vi "CRYResize Panel Child For Load.vi"(8 "spliter array":refnum<vi>[](array[refnum]), 9 "SubPanel array":refnum<vi>[](array[refnum]), 10 "DataView Array Idx":i32) -> ()   [LabVIEW 2013]
uses:
  CRYNew View Global.vi
panel:
  in  "cur_sp_hei":i32
  in  "cur_sp_wid":i32
  in  "cur_sp_ypos":i32
  in  "cur_sp_xpos":i32
  in  "sp_mUp_hei":i32
  in  "sp_mUp_wid":i32
  in  "sp_mUp_ypos":i32
  in  "sp_mUp_xpos":i32
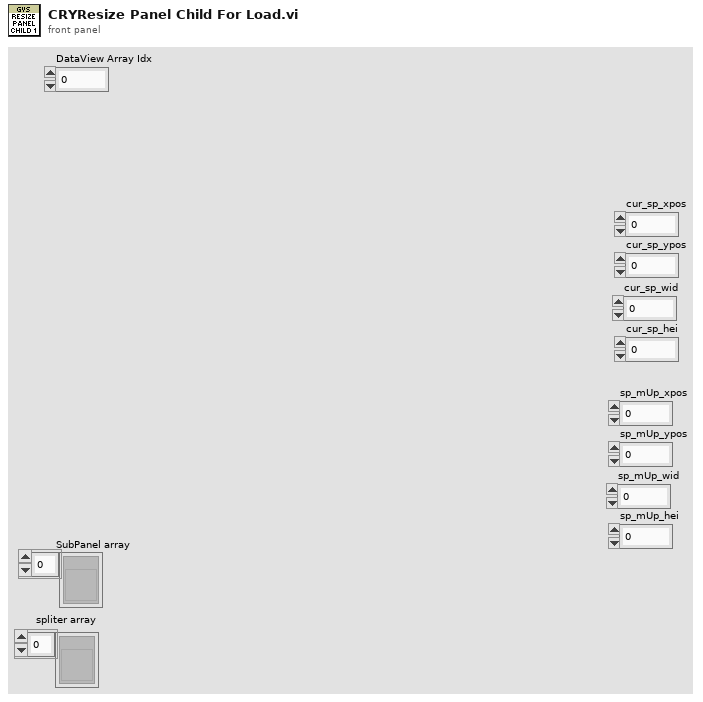
[diagram p1: front panel]
types:
  T1 = typedef "Graph Main Info Cluster.ctl" = cluster{"Selected_BarIdx":i32, "Selected_PanelIdx":i32, "Graph Main VIRef":refnum<vi>, "ToolBarClick":bool, "Spliter Ref Array":refnum<vi>[], "Panel Ref Array":refnum<vi>[], "Spliter_matrix":i32[][], "Panel_matrix":i32[][], "child_spliterIdx_matrix":i32[][], "split_pos_matrix":i32[][], "Title State":bool, "sQueueName":string, "Frame nID":i32, "Graph VIRef Array":cluster{"Graph VIRef":refnum<vi>, "Panel Idx":i32, "Frame VIRef":refnum<vi>, "Icon Ring":i32, "Graph Type":string}[], "View Type":string}
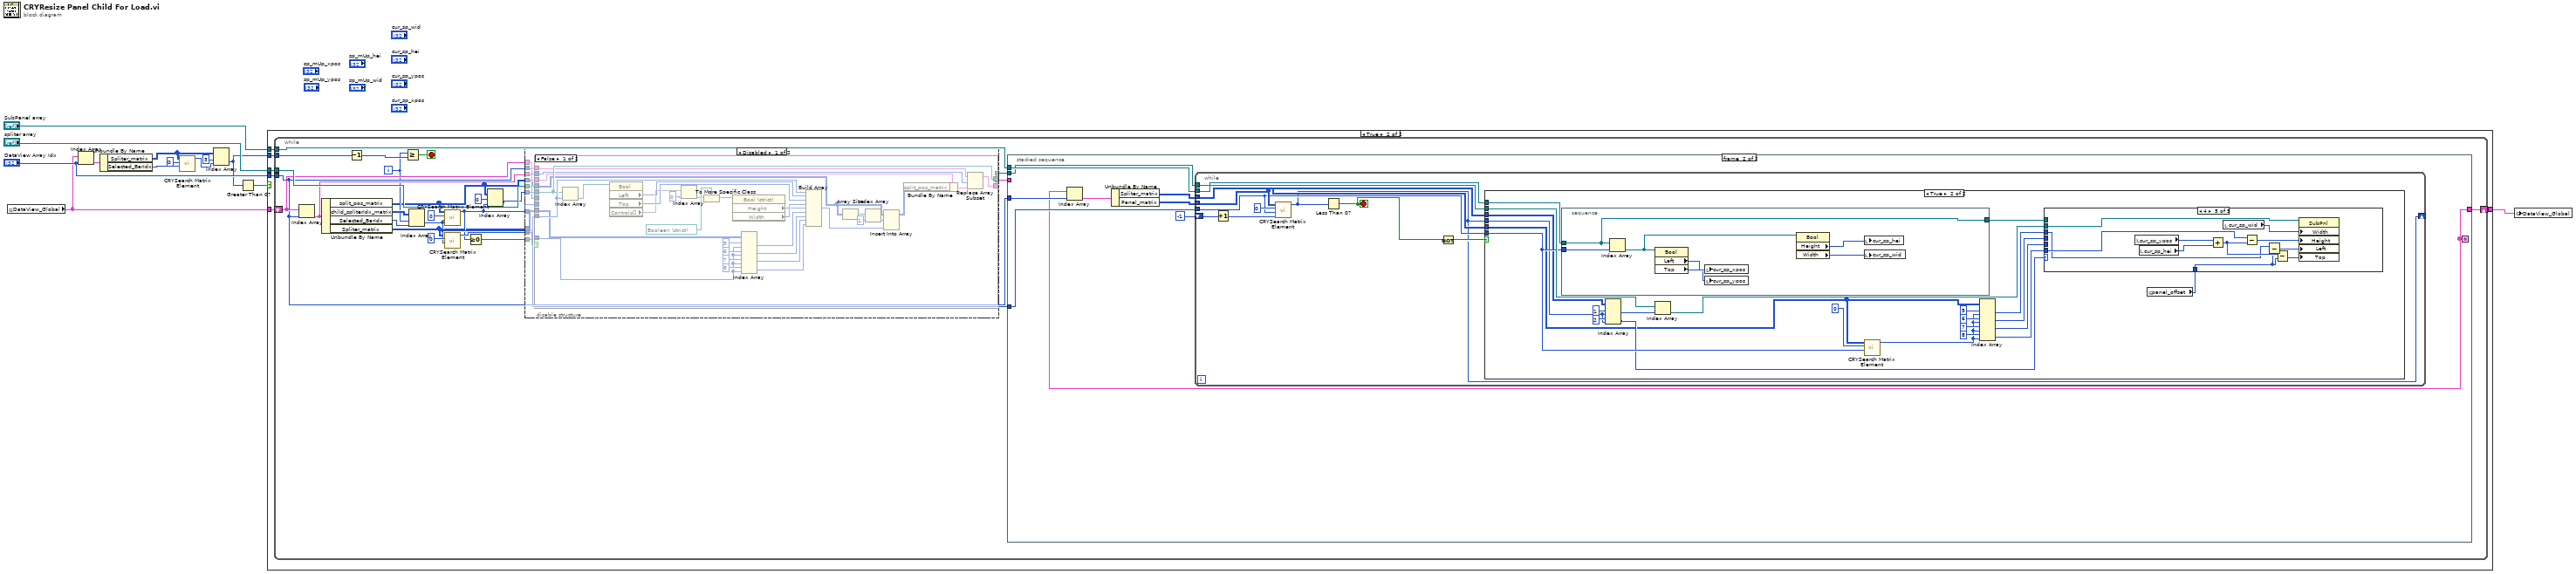
[diagram p0: block diagram]
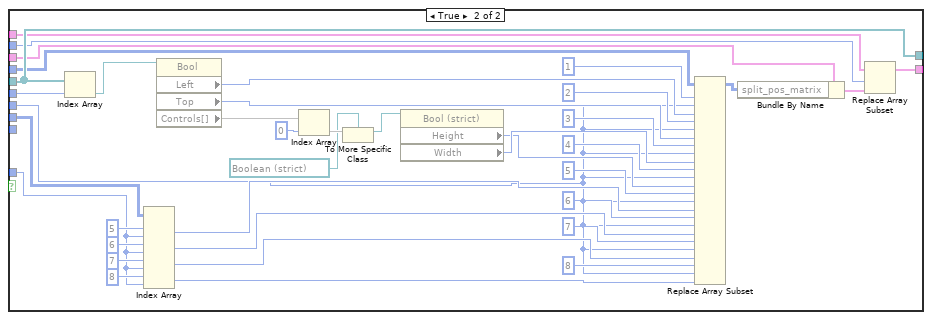
[diagram p3: hidden frame]
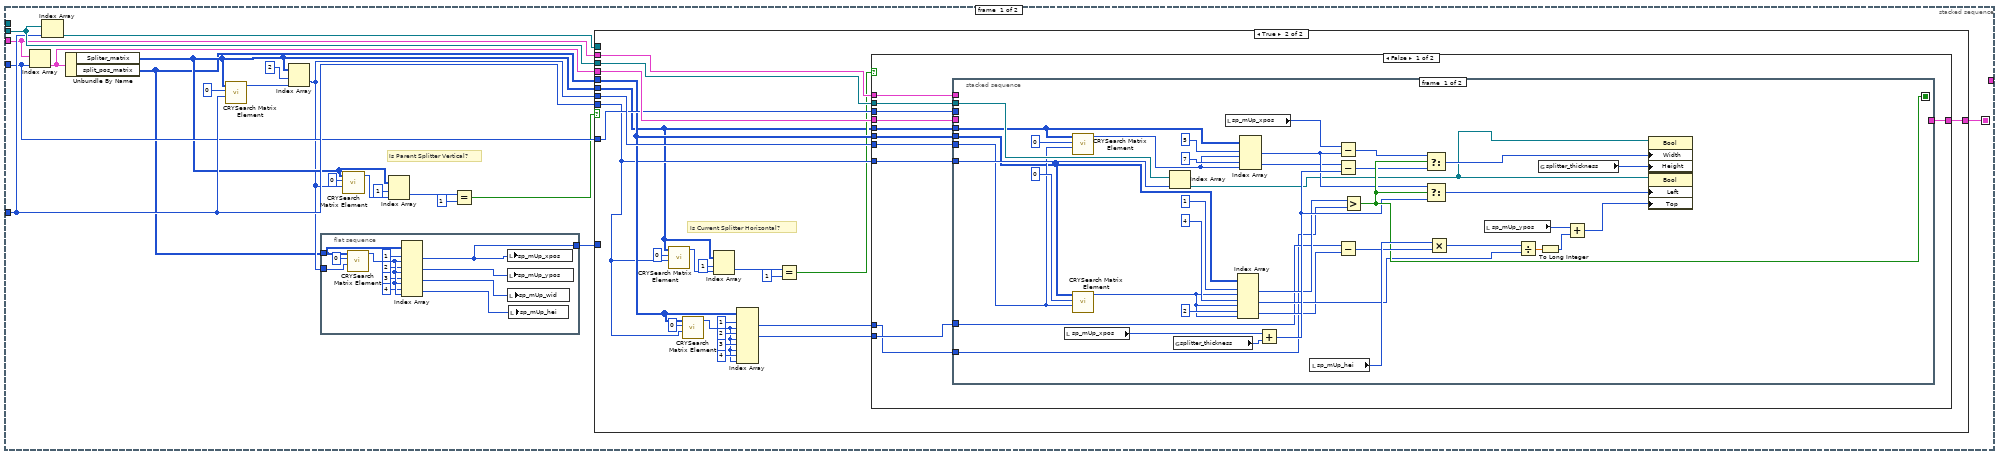
[diagram p5: hidden frame]
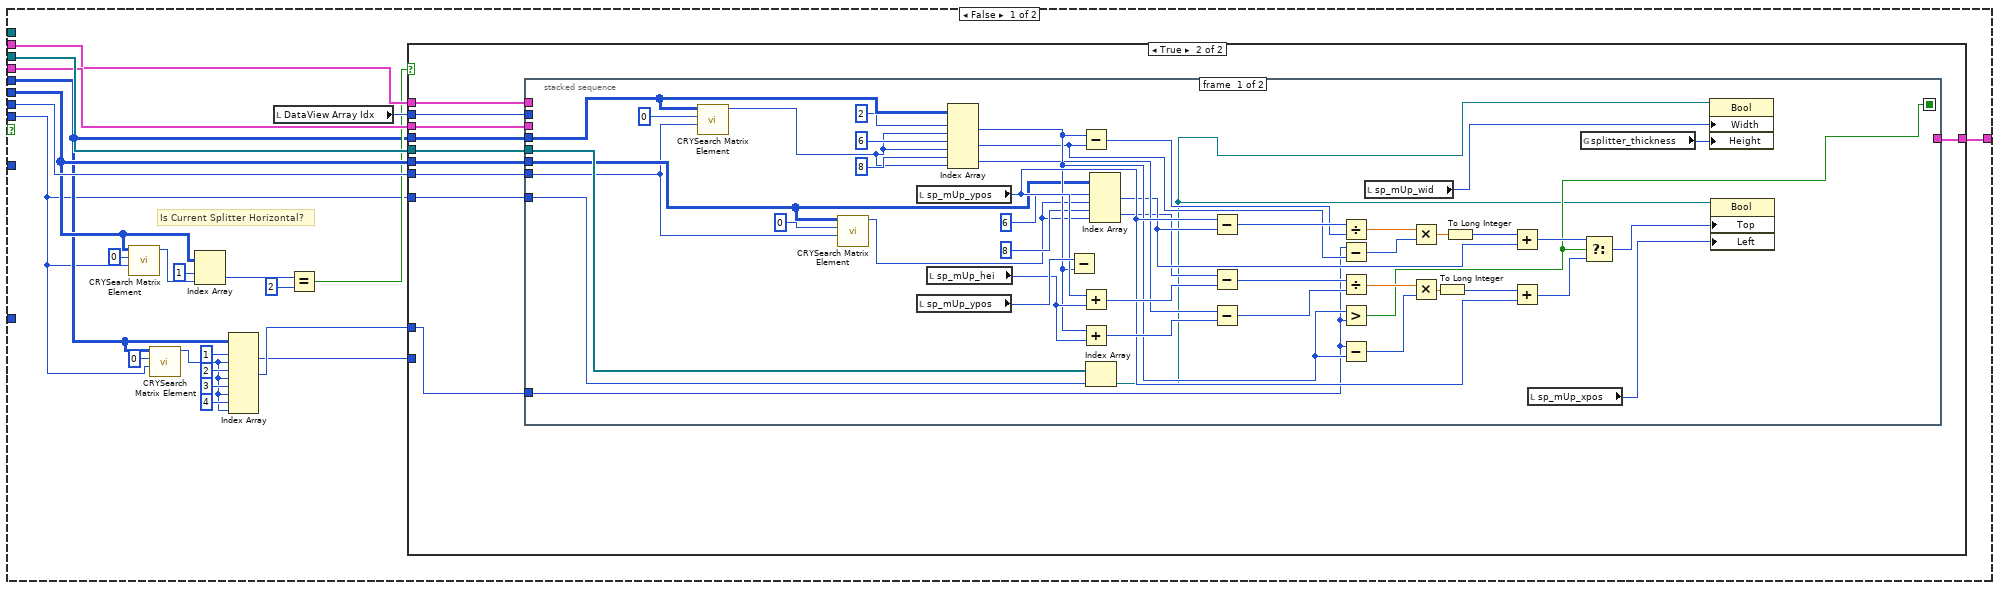
[diagram p6: hidden frame]
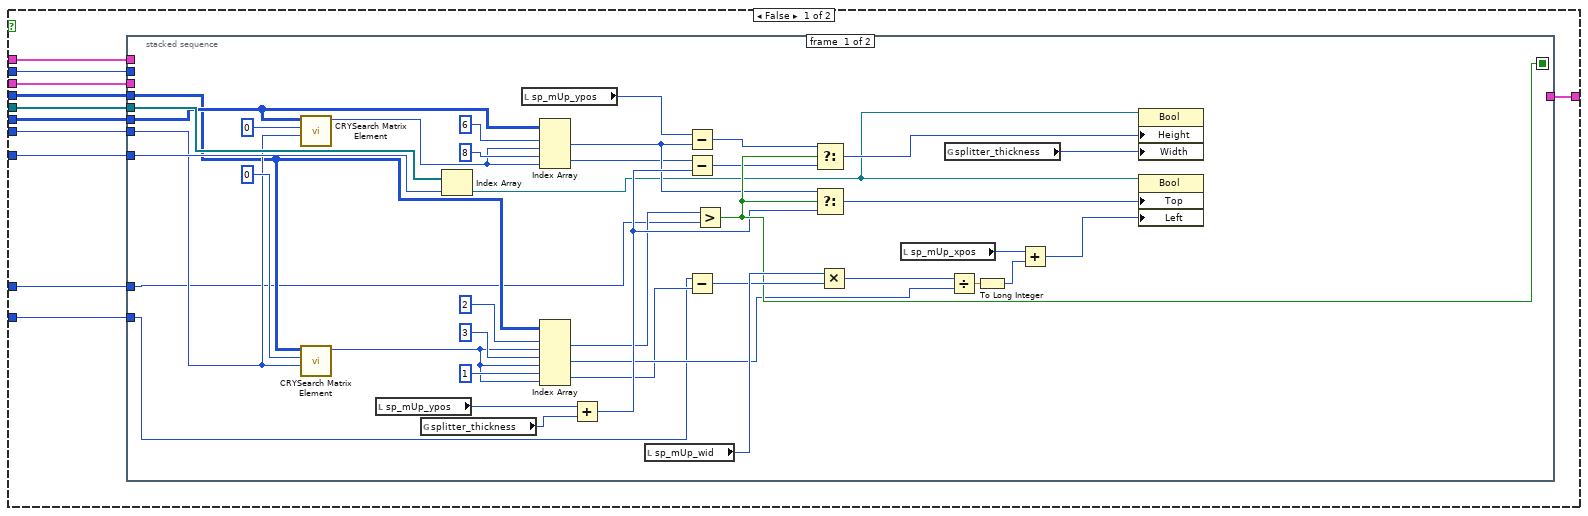
[diagram p7: hidden frame]
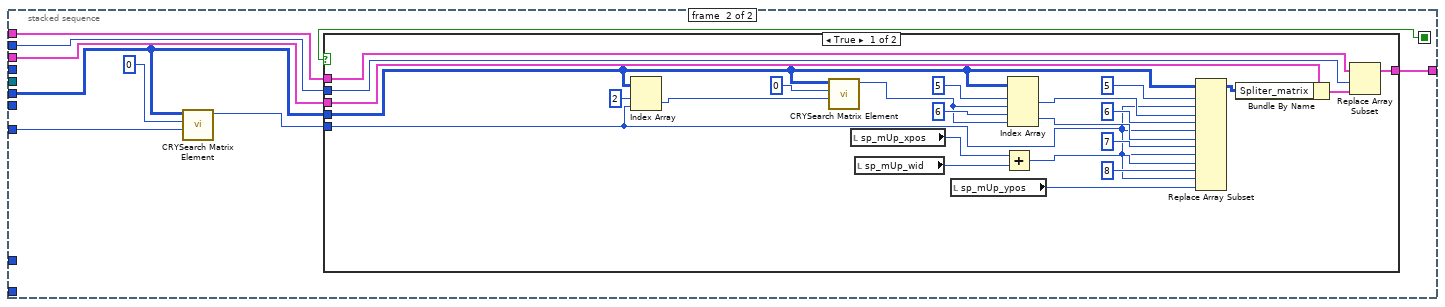
[diagram p8: hidden frame]
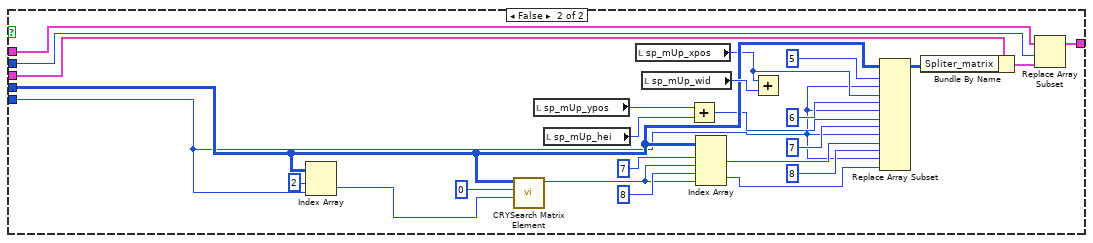
[diagram p9: hidden frame]
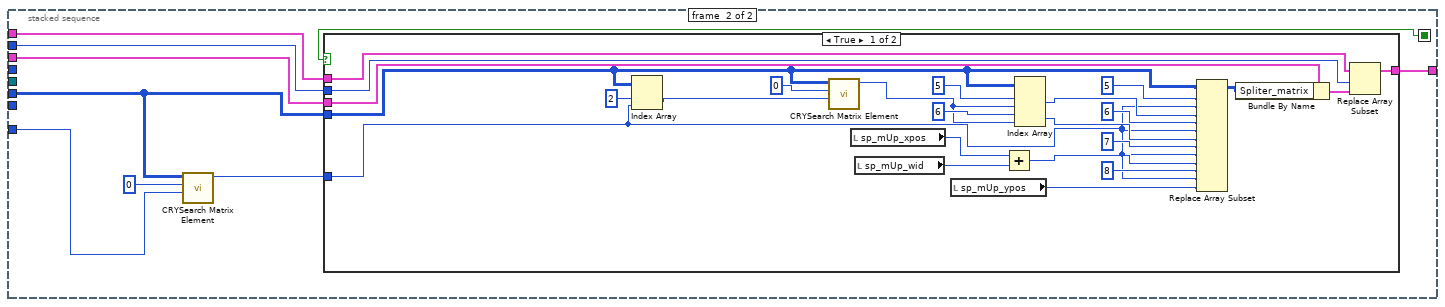
[diagram p10: hidden frame]
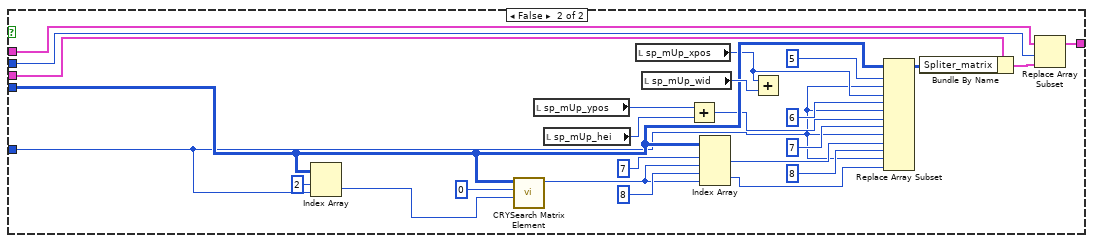
[diagram p11: hidden frame]
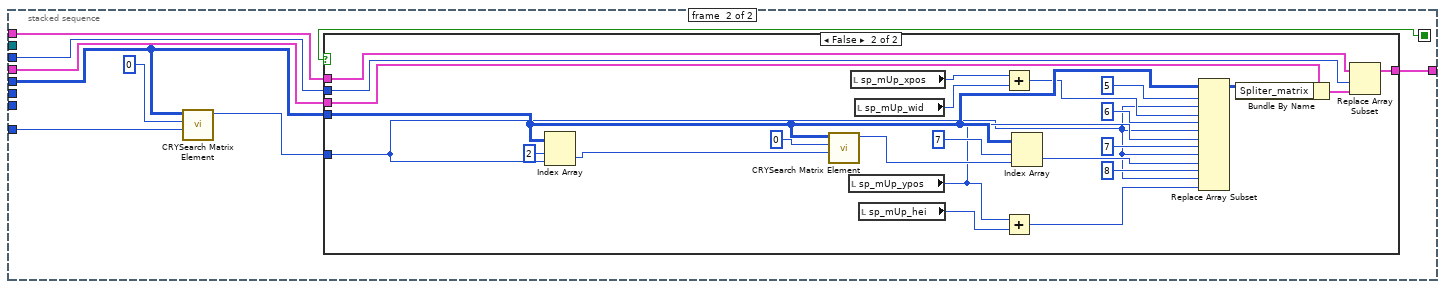
[diagram p12: hidden frame]
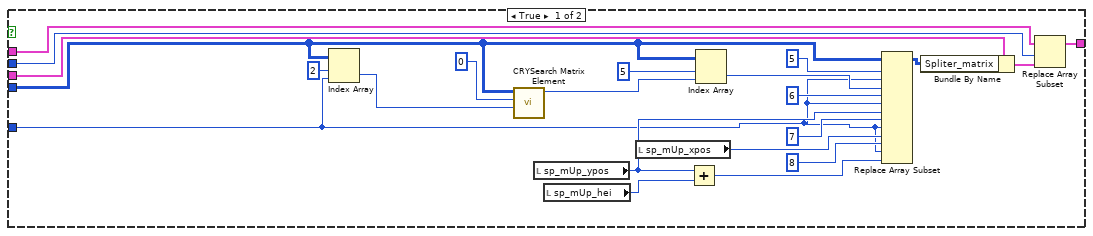
[diagram p13: hidden frame]
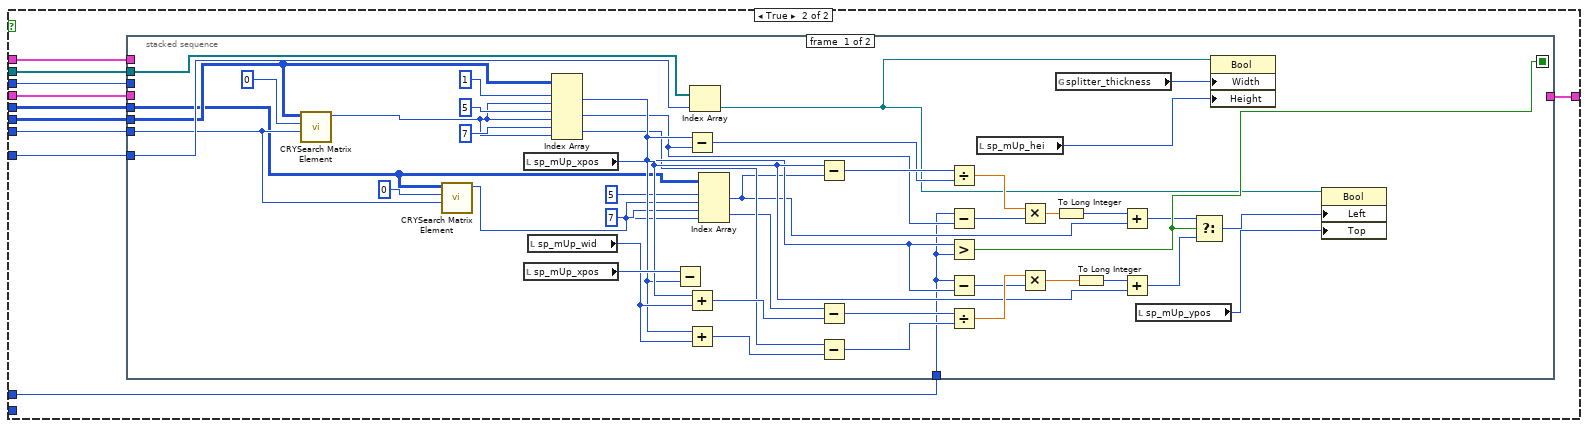
[diagram p14: hidden frame]
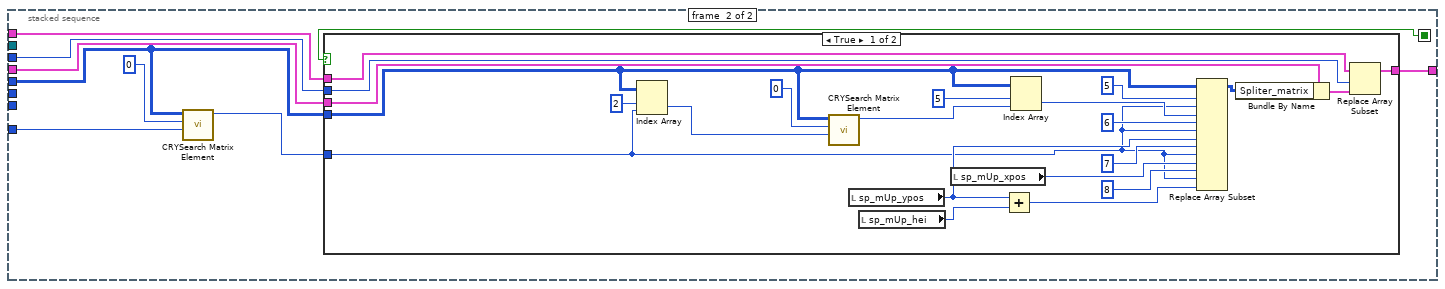
[diagram p15: hidden frame]
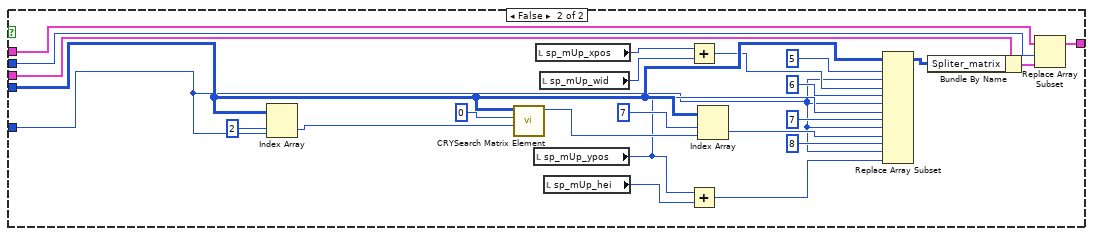
[diagram p16: hidden frame]
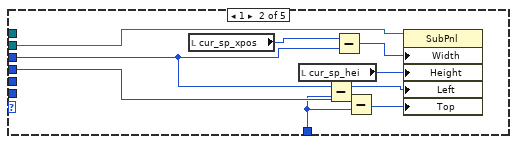
[diagram p19: hidden frame]
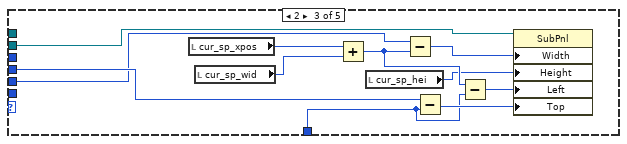
[diagram p20: hidden frame]
diagram:
  n1 = global read "CRYNew View Global.vi" "DataView_Global"() -> (w7:T1[])
  n2 = Index Array(array=w7, index="DataView Array Idx") -> (element=w10:T1)
  n3 = Unbundle By Name(w10) -> ("Spliter_matrix"=w4:i32[][], "Selected_BarIdx"=w9:i32)
  n4 = call "CRYSearch Matrix Element.vi"("element"=w9, "index (row)"=0, "matrix in"=w4) -> ("index of element"=w2:i32)  [unwired: 8 in]
  n5 = Index Array(array=w4, index (row)=3, index (col)=w2) -> (element=w1:i32)
  n6 = Greater Than 0?(x=w1) -> (x > 0?=w5:bool)
  n7 = case shown="True" w5 {
    tunnel: "spliter array" -> [_ w20]
    tunnel: "SubPanel array" -> [_ w19]
    tunnel: "DataView Array Idx" -> [_ w18]
    tunnel: w1 -> [_ w17]
    tunnel: w7 -> [w14 w16]
    tunnel: [w14 w15] -> w6
    frame False {
    }
    frame True {
      n8 = while {
        tunnel: w20 -> [w41]
        tunnel: w17 -> [w30]
        tunnel: w19 -> [w39]
        tunnel: w18 -> [w31]
        shift-right: [w32] -> w15
        shift-left: w16 -> [w34]
        i -> [w28]
        stop <- w42 stop-if-true
        n9 = Index Array(array=w34, index=w31) -> (element=w38:T1)
        n10 = Unbundle By Name(w38) -> ("split_pos_matrix"=w24:i32[][], "child_spliterIdx_matrix"=w29:i32[][], "Selected_BarIdx"=w27:i32, "Spliter_matrix"=w21:i32[][])
        n11 = Decrement(x=w30) -> (x-1=w43:i32)
        n12 = Greater Or Equal?(x=w28, y=w43) -> (x >= y?=w42:bool)
        n13 = Index Array(array=w29, index (row)=w28, index (col)=w27) -> (element=w26:i32)
        n14 = call "CRYSearch Matrix Element.vi"("element"=w26, "index (row)"=0, "matrix in"=w24) -> ("index of element"=w23:i32)  [unwired: 8 in]
        n15 = call "CRYSearch Matrix Element.vi"("element"=w26, "index (row)"=0, "matrix in"=w21) -> ("index of element"=w36:i32)  [unwired: 8 in]
        n16 = Greater Or Equal To 0?(x=w23) -> (x >= 0?=w44:bool)
        n17 = Index Array(array=w24, index (row)=0, index (col)=w23) -> (element=w22:i32)
        n18 = disable-structure shown="Disabled" {
          disable-tunnel: w44 -> [w57 _]
          disable-tunnel: w41 -> [w56 w129]
          disable-tunnel: [w55 w129] -> w40
          disable-tunnel: w38 -> [w54 _]
          disable-tunnel: w36 -> [w53 _]
          disable-tunnel: w34 -> [w52 w130]
          disable-tunnel: [w51 w130] -> w33
          disable-tunnel: w31 -> [w50 _]
          disable-tunnel: w26 -> [w49 _]
          disable-tunnel: w24 -> [w48 _]
          disable-tunnel: w23 -> [w47 _]
          disable-tunnel: w22 -> [w46 _]
          disable-tunnel: w21 -> [w45 _]
          frame Disabled {
            n19 = case shown="False" w57 {
              tunnel: w47 -> [_ w93]
              tunnel: w49 -> [w90 _]
              tunnel: w56 -> [w79 w121]
              tunnel: w46 -> [_ w127]
              tunnel: [w79 w121] -> w55
              tunnel: w53 -> [w69 w110]
              tunnel: w45 -> [w68 w111]
              tunnel: w48 -> [w60 w109]
              tunnel: w50 -> [w77 w119]
              tunnel: w54 -> [w76 w118]
              tunnel: w52 -> [w75 w117]
              tunnel: [w74 w116] -> w51
              frame False {
                n20 = Index Array(array=w79, index=w90) -> (element=w89:refnum<vi>)
                n21 = property class="Bool"(reference=w89) -> ("Left"=w88:i32, "Top"=w87:i32, "Controls[]"=w86)  [unwired: 1 in, 2 out]
                n22 = Index Array(array=w86, index=0) -> (element=w84)
                n23 = To More Specific Class(target class=refnum<vi> refnum ("Boolean"), reference=w84) -> (specific class reference=w82:refnum<vi>)  [unwired: 1 in, 1 out]
                n24 = property class="Bool (strict)"(reference=w82) -> ("Height"=w80:u32, "Width"=w81:u32)  [unwired: 1 in, 2 out]
                n25 = Index Array(array=w68, index (row) #1=5 ("index (row)"), index (col) #1=w69, index (row) #2=6 ("index (row)"), index (col) #2=w69, index (row) #3=7 ("index (row)"), index (col) #3=w69, index (row) #4=8 ("index (row)"), index (col) #4=w69) -> (element #1=w67:i32, element #2=w66:i32, element #3=w65:i32, element #4=w64:i32)
                n26 = Build Array(w90, w88, w87, w81, w80, w67, w66, w65, w64) -> (w59:u32[])
                n27 = Array Size(array=w60) -> (size(s)=w63:i32[])
                n28 = Index Array(array=w63, index=1) -> (element=w61:i32)
                n29 = Insert Into Array(array=w60, index (col)=w61, new element=w59) -> (w58:i32[][])  [unwired: 1 in]
                n30 = Bundle By Name(cluster=w76, "split_pos_matrix"=w58) -> (w78:T1)
                n31 = Replace Array Subset(array=w75, new element=w78, index=w77) -> (w74:T1[])
              }
              frame True {
                n32 = Index Array(array=w121, index=w127) -> (element=w128:refnum<vi>)
                n33 = Index Array(array=w111, index (row) #1=5 ("index (row)"), index (col) #1=w110, index (row) #2=6 ("index (row)"), index (col) #2=w110, index (row) #3=7 ("index (row)"), index (col) #3=w110, index (row) #4=8 ("index (row)"), index (col) #4=w110) -> (element #1=w99:i32, element #2=w97:i32, element #3=w95:i32, element #4=w92:i32)
                n34 = property class="Bool"(reference=w128) -> ("Left"=w107:i32, "Top"=w105:i32, "Controls[]"=w126)  [unwired: 1 in, 2 out]
                n35 = Index Array(array=w126, index=0) -> (element=w124)
                n36 = To More Specific Class(target class=refnum<vi> refnum ("Boolean"), reference=w124) -> (specific class reference=w122:refnum<vi>)  [unwired: 1 in, 1 out]
                n37 = property class="Bool (strict)"(reference=w122) -> ("Height"=w101:u32, "Width"=w103:u32)  [unwired: 1 in, 2 out]
                n38 = Replace Array Subset(array=w109, new element #1=w107, index (row) #1=1 ("disabled index (row)"), index (col) #1=w93, new element #2=w105, index (row) #2=2 ("disabled index (row)"), index (col) #2=w93, new element #3=w103, index (row) #3=3 ("disabled index (row)"), index (col) #3=w93, new element #4=w101, index (row) #4=4 ("disabled index (row)"), index (col) #4=w93, new element #5=w99, index (row) #5=5 ("disabled index (row)"), index (col) #5=w93, new element #6=w97, index (row) #6=6 ("disabled index (row)"), index (col) #6=w93, new element #7=w95, index (row) #7=7 ("disabled index (row)"), index (col) #7=w93, new element #8=w92, index (row) #8=8 ("disabled index (row)"), index (col) #8=w93) -> (w91:i32[][])
                n39 = Bundle By Name(cluster=w118, "split_pos_matrix"=w91) -> (w120:T1)
                n40 = Replace Array Subset(array=w117, new element=w120, index=w119) -> (w116:T1[])
              }
            }
          }
          frame Enabled {
          }
        }
        n41 = stacked-sequence {
          seq-local: [w144 _] -> [_ w645]
          tunnel: w40 -> [w149 w651]
          tunnel: w26 -> [w146 w653]
          tunnel: w39 -> [_ w652]
          tunnel: w31 -> [w143 w648]
          tunnel: w33 -> [w145 _]
          tunnel: [_ w645] -> w32
          frame #0 {
            # "Is Parent Splitter Vertical?"
            n42 = Index Array(array=w145, index=w143) -> (element=w148:T1)
            n43 = Index Array(array=w149, index=w146) -> (element=w150:refnum<vi>)
            n44 = Unbundle By Name(w148) -> ("Spliter_matrix"=w139:i32[][], "split_pos_matrix"=w132:i32[][])
            n45 = call "CRYSearch Matrix Element.vi"("element"=w146, "index (row)"=0, "matrix in"=w139) -> ("index of element"=w141:i32)  [unwired: 8 in]
            n46 = Index Array(array=w139, index (row)=2, index (col)=w141) -> (element=w133:i32)
            n47 = flat-sequence {
              tunnel: w133 -> [w161]
              tunnel: w132 -> [w152]
              tunnel: [w151] -> w131
              frame #0 {
                n48 = call "CRYSearch Matrix Element.vi"("element"=w161, "index (row)"=0, "matrix in"=w152) -> ("index of element"=w160:i32)  [unwired: 8 in]
                n49 = Index Array(array=w152, index (row) #1=1 ("disabled index (row)"), index (col) #1=w160, index (row) #2=2 ("disabled index (row)"), index (col) #2=w160, index (row) #3=3 ("disabled index (row)"), index (col) #3=w160, index (row) #4=4 ("disabled index (row)"), index (col) #4=w160) -> (element #1=w151:i32, element #2=w155:i32, element #3=w154:i32, element #4=w153:i32)
                n50 = local write "sp_mUp_xpos"(w151) -> ()
                n51 = local write "sp_mUp_ypos"(w155) -> ()
                n52 = local write "sp_mUp_wid"(w154) -> ()
                n53 = local write "sp_mUp_hei"(w153) -> ()
              }
            }
            n54 = call "CRYSearch Matrix Element.vi"("element"=w133, "index (row)"=0, "matrix in"=w139) -> ("index of element"=w134:i32)  [unwired: 8 in]
            n55 = Index Array(array=w139, index (row)=1 ("disabled index (row)"), index (col)=w134) -> (element=w137:i32)
            n56 = Equal?(x=w137, y=1) -> (x = y?=w135:bool)
            n57 = case shown="True" w135 {
              tunnel: w150 -> [_ _]
              tunnel: w133 -> [w185 w429]
              tunnel: w149 -> [w184 w428]
              tunnel: w146 -> [w163 w411]
              tunnel: w132 -> [w166 w412]
              tunnel: w139 -> [w174 w407]
              tunnel: w148 -> [w183 w427]
              tunnel: w145 -> [w181 w426]
              tunnel: [w180 w425] -> w144
              tunnel: w143 -> [_ w424]
              tunnel: w131 -> [_ _]
              frame False {
                # "Is Current Splitter Horizontal?"
                n58 = call "CRYSearch Matrix Element.vi"("element"=w163, "index (row)"=0, "matrix in"=w174) -> ("index of element"=w179:i32)  [unwired: 8 in]
                n59 = call "CRYSearch Matrix Element.vi"("element"=w163, "index (row)"=0, "matrix in"=w166) -> ("index of element"=w168:i32)  [unwired: 8 in]
                n60 = Index Array(array=w174, index (row)=1 ("disabled index (row)"), index (col)=w179) -> (element=w177:i32)
                n61 = Index Array(array=w166, index (row) #1=1 ("disabled index (row)"), index (col) #1=w168, index (row) #2=2 ("disabled index (row)"), index (col) #2=w168, index (row) #3=3 ("disabled index (row)"), index (col) #3=w168, index (row) #4=4 ("disabled index (row)"), index (col) #4=w168) -> (element #1=w164:i32, element #2=w165:i32)  [unwired: 2 out]
                n62 = local read "DataView Array Idx"() -> (w182:i32)
                n63 = Equal?(x=w177, y=2) -> (x = y?=w173:bool)
                n64 = case shown="True" w173 {
                  tunnel: w185 -> [w194 w301]
                  tunnel: w184 -> [w196 w302]
                  tunnel: w163 -> [w195 w303]
                  tunnel: w166 -> [w193 w300]
                  tunnel: w174 -> [w192 w299]
                  tunnel: w183 -> [w191 w298]
                  tunnel: w182 -> [w190 w297]
                  tunnel: w181 -> [w189 w296]
                  tunnel: [w188 w295] -> w180
                  tunnel: w165 -> [w187 w294]
                  tunnel: w164 -> [w186 _]
                  frame False {
                    n65 = stacked-sequence {
                      seq-local: [w224 _] -> [_ w244]
                      tunnel: w196 -> [w235 _]
                      tunnel: w195 -> [w234 w239]
                      tunnel: w194 -> [w217 _]
                      tunnel: w193 -> [w210 _]
                      tunnel: w192 -> [w216 w241]
                      tunnel: w191 -> [_ w243]
                      tunnel: w190 -> [_ w242]
                      tunnel: w189 -> [_ w237]
                      tunnel: [_ w236] -> w188
                      tunnel: w187 -> [w202 _]
                      tunnel: w186 -> [w201 _]
                      frame #0 {
                        n66 = call "CRYSearch Matrix Element.vi"("element"=w217, "index (row)"=0, "matrix in"=w216) -> ("index of element"=w213:i32)  [unwired: 8 in]
                        n67 = call "CRYSearch Matrix Element.vi"("element"=w217, "index (row)"=0, "matrix in"=w210) -> ("index of element"=w206:i32)  [unwired: 8 in]
                        n68 = local read "sp_mUp_ypos"() -> (w233:i32)
                        n69 = global read "CRYNew View Global.vi" "splitter_thickness"() -> (w197:u32)
                        n70 = Index Array(array=w235, index=w234) -> (element=w200:refnum<vi>)
                        n71 = local read "sp_mUp_ypos"() -> (w223:i32)
                        n72 = Index Array(array=w216, index (row) #1=6 ("index (row)"), index (col) #1=w213, index (row) #2=8 ("index (row)"), index (col) #2=w213) -> (element #1=w212:i32, element #2=w211:i32)
                        n73 = Index Array(array=w210, index (row) #1=2 ("index (row)"), index (col) #1=w206, index (row) #2=3 ("index (row)"), index (col) #2=w206, index (row) #3=1 ("index (row)"), index (col) #3=w206) -> (element #1=w205:i32, element #2=w204:i32, element #3=w203:i32)
                        n74 = Add(x=w233, y=w197) -> (x+y=w221:u32)
                        n75 = local read "sp_mUp_wid"() -> (w230:i32)
                        n76 = Subtract(x=w223, y=w212) -> (x-y=w222:i32)
                        n77 = Subtract(x=w211, y=w221) -> (x-y=w220:u32)
                        n78 = Subtract(x=w201, y=w203) -> (x-y=w225:i32)
                        n79 = Greater?(x=w205, y=w202) -> (0:w224:bool)
                        n80 = Select(t=w222, s=w224, f=w220) -> (s? t:f=w231:u32)
                        n81 = Select(t=w212, s=w224, f=w221) -> (s? t:f=w232:u32)
                        n82 = Multiply(x=w230, y=w225) -> (x*y=w229:i32)
                        n83 = local read "sp_mUp_xpos"() -> (w228:i32)
                        n84 = global read "CRYNew View Global.vi" "splitter_thickness"() -> (w199:u32)
                        n85 = Divide(x=w229, y=w204) -> (x/y=w227:dbl)
                        n86 = To Long Integer(number=w227) -> (32bit integer=w198:i32)
                        n87 = Add(x=w228, y=w198) -> (x+y=w226:i32)
                        n88 = property class="Bool"(reference=w200, "Height"=w231, "Width"=w199) -> ()  [unwired: 1 in, 2 out]
                        n89 = property class="Bool"(reference=w200, "Top"=w232, "Left"=w226) -> ()  [unwired: 1 in, 2 out]
                      }
                      frame #1 {
                        n90 = call "CRYSearch Matrix Element.vi"("element"=w239, "index (row)"=0, "matrix in"=w241) -> ("index of element"=w238:i32)  [unwired: 8 in]
                        n91 = case shown="True" w244 {
                          tunnel: w238 -> [w247 w271]
                          tunnel: w241 -> [w255 w279]
                          tunnel: w243 -> [w265 w289]
                          tunnel: w242 -> [w264 w288]
                          tunnel: w237 -> [w262 w286]
                          tunnel: [w261 w285] -> w236
                          frame True {
                            n92 = Index Array(array=w255, index (row)=2, index (col)=w247) -> (element=w259:i32)
                            n93 = call "CRYSearch Matrix Element.vi"("element"=w259, "index (row)"=0, "matrix in"=w255) -> ("index of element"=w256:i32)  [unwired: 8 in]
                            n94 = local read "sp_mUp_xpos"() -> (w267:i32)
                            n95 = local read "sp_mUp_wid"() -> (w268:i32)
                            n96 = local read "sp_mUp_ypos"() -> (w246:i32)
                            n97 = Add(x=w267, y=w268) -> (x+y=w249:i32)
                            n98 = Index Array(array=w255, index (row) #1=5 ("index (row)"), index (col) #1=w256, index (row) #2=6 ("index (row)"), index (col) #2=w256) -> (element #1=w253:i32, element #2=w251:i32)
                            n99 = Replace Array Subset(array=w255, new element #1=w253, index (row) #1=5 ("disabled index (row)"), index (col) #1=w247, new element #2=w251, index (row) #2=6 ("disabled index (row)"), index (col) #2=w247, new element #3=w249, index (row) #3=7 ("disabled index (row)"), index (col) #3=w247, new element #4=w246, index (row) #4=8 ("disabled index (row)"), index (col) #4=w247) -> (w245:i32[][])
                            n100 = Bundle By Name(cluster=w265, "Spliter_matrix"=w245) -> (w266:T1)
                            n101 = Replace Array Subset(array=w262, new element=w266, index=w264) -> (w261:T1[])
                          }
                          frame False {
                            n102 = Index Array(array=w279, index (row)=2, index (col)=w271) -> (element=w283:i32)
                            n103 = call "CRYSearch Matrix Element.vi"("element"=w283, "index (row)"=0, "matrix in"=w279) -> ("index of element"=w280:i32)  [unwired: 8 in]
                            n104 = local read "sp_mUp_ypos"() -> (w292:i32)
                            n105 = local read "sp_mUp_hei"() -> (w293:i32)
                            n106 = local read "sp_mUp_xpos"() -> (w277:i32)
                            n107 = local read "sp_mUp_wid"() -> (w291:i32)
                            n108 = Add(x=w292, y=w293) -> (x+y=w275:i32)
                            n109 = Index Array(array=w279, index (row) #1=7 ("index (row)"), index (col) #1=w280, index (row) #2=8 ("index (row)"), index (col) #2=w280) -> (element #1=w273:i32, element #2=w270:i32)
                            n110 = Add(x=w277, y=w291) -> ()  [unwired: 1 out]
                            n111 = Replace Array Subset(array=w279, new element #1=w277, index (row) #1=5 ("disabled index (row)"), index (col) #1=w271, new element #2=w275, index (row) #2=6 ("disabled index (row)"), index (col) #2=w271, new element #3=w273, index (row) #3=7 ("disabled index (row)"), index (col) #3=w271, new element #4=w270, index (row) #4=8 ("disabled index (row)"), index (col) #4=w271) -> (w269:i32[][])
                            n112 = Bundle By Name(cluster=w289, "Spliter_matrix"=w269) -> (w290:T1)
                            n113 = Replace Array Subset(array=w286, new element=w290, index=w288) -> (w285:T1[])
                          }
                        }
                      }
                    }
                  }
                  frame True {
                    n114 = stacked-sequence {
                      seq-local: [w327 _] -> [_ w357]
                      tunnel: w303 -> [w310 w353]
                      tunnel: w302 -> [w347 _]
                      tunnel: w301 -> [w308 _]
                      tunnel: w300 -> [w324 _]
                      tunnel: w299 -> [w316 w352]
                      tunnel: w298 -> [_ w356]
                      tunnel: w297 -> [_ w355]
                      tunnel: w296 -> [_ w350]
                      tunnel: [_ w349] -> w295
                      tunnel: w294 -> [w309 _]
                      frame #0 {
                        n115 = call "CRYSearch Matrix Element.vi"("element"=w308, "index (row)"=0, "matrix in"=w324) -> ("index of element"=w320:i32)  [unwired: 8 in]
                        n116 = call "CRYSearch Matrix Element.vi"("element"=w308, "index (row)"=0, "matrix in"=w316) -> ("index of element"=w313:i32)  [unwired: 8 in]
                        n117 = local read "sp_mUp_ypos"() -> (w331:i32)
                        n118 = local read "sp_mUp_ypos"() -> (w348:i32)
                        n119 = local read "sp_mUp_hei"() -> (w344:i32)
                        n120 = Index Array(array=w324, index (row) #1=2 ("index (row)"), index (col) #1=w320, index (row) #2=6 ("index (row)"), index (col) #2=w320, index (row) #3=8 ("index (row)"), index (col) #3=w320) -> (element #1=w319:i32, element #2=w318:i32, element #3=w317:i32)
                        n121 = Subtract(x=w348, y=w319) -> ()  [unwired: 1 out]
                        n122 = Subtract(x=w319, y=w318) -> (x-y=w338:i32)
                        n123 = Add(x=w331, y=w344) -> (x+y=w332:i32)
                        n124 = Add(x=w319, y=w344) -> (x+y=w333:i32)
                        n125 = Index Array(array=w347, index=w310) -> (element=w307:refnum<vi>)
                        n126 = Index Array(array=w316, index (row) #1=6 ("index (row)"), index (col) #1=w313, index (row) #2=8 ("index (row)"), index (col) #2=w313) -> (element #1=w312:i32, element #2=w311:i32)
                        n127 = Subtract(x=w331, y=w312) -> (x-y=w339:i32)
                        n128 = Subtract(x=w311, y=w332) -> (x-y=w343:i32)
                        n129 = Subtract(x=w317, y=w333) -> (x-y=w342:i32)
                        n130 = Divide(x=w339, y=w338) -> (x/y=w337:dbl)
                        n131 = Subtract(x=w309, y=w318) -> (x-y=w336:i32)
                        n132 = Divide(x=w343, y=w342) -> (x/y=w341:dbl)
                        n133 = Greater?(x=w319, y=w309) -> (0:w327:bool)
                        n134 = Subtract(x=w309, y=w319) -> (x-y=w334:i32)
                        n135 = local read "sp_mUp_wid"() -> (w346:i32)
                        n136 = Multiply(x=w337, y=w336) -> (x*y=w335:dbl)
                        n137 = Multiply(x=w341, y=w334) -> (x*y=w340:dbl)
                        n138 = To Long Integer(number=w340) -> (32bit integer=w305:i32)
                        n139 = To Long Integer(number=w335) -> (32bit integer=w306:i32)
                        n140 = Add(x=w306, y=w312) -> (x+y=w330:i32)
                        n141 = Add(x=w305, y=w331) -> (x+y=w329:i32)
                        n142 = local read "sp_mUp_xpos"() -> (w345:i32)
                        n143 = global read "CRYNew View Global.vi" "splitter_thickness"() -> (w304:u32)
                        n144 = Select(t=w330, s=w327, f=w329) -> (s? t:f=w328:i32)
                        n145 = property class="Bool"(reference=w307, "Width"=w346, "Height"=w304) -> ()  [unwired: 1 in, 2 out]
                        n146 = property class="Bool"(reference=w307, "Top"=w328, "Left"=w345) -> ()  [unwired: 1 in, 2 out]
                      }
                      frame #1 {
                        n147 = call "CRYSearch Matrix Element.vi"("element"=w353, "index (row)"=0, "matrix in"=w352) -> ("index of element"=w351:i32)  [unwired: 8 in]
                        n148 = case shown="True" w357 {
                          tunnel: w351 -> [w359 w383]
                          tunnel: w352 -> [w368 w392]
                          tunnel: w356 -> [w378 w402]
                          tunnel: w355 -> [w377 w401]
                          tunnel: w350 -> [w375 w399]
                          tunnel: [w374 w398] -> w349
                          frame True {
                            n149 = Index Array(array=w368, index (row)=2, index (col)=w359) -> (element=w373:i32)
                            n150 = call "CRYSearch Matrix Element.vi"("element"=w373, "index (row)"=0, "matrix in"=w368) -> ("index of element"=w369:i32)  [unwired: 8 in]
                            n151 = local read "sp_mUp_xpos"() -> (w380:i32)
                            n152 = local read "sp_mUp_wid"() -> (w381:i32)
                            n153 = local read "sp_mUp_ypos"() -> (w358:i32)
                            n154 = Add(x=w380, y=w381) -> (x+y=w361:i32)
                            n155 = Index Array(array=w368, index (row) #1=5 ("index (row)"), index (col) #1=w369, index (row) #2=6 ("index (row)"), index (col) #2=w369) -> (element #1=w365:i32, element #2=w363:i32)
                            n156 = Replace Array Subset(array=w368, new element #1=w365, index (row) #1=5 ("disabled index (row)"), index (col) #1=w359, new element #2=w363, index (row) #2=6 ("disabled index (row)"), index (col) #2=w359, new element #3=w361, index (row) #3=7 ("disabled index (row)"), index (col) #3=w359, new element #4=w358, index (row) #4=8 ("disabled index (row)"), index (col) #4=w359) -> (w367:i32[][])
                            n157 = Bundle By Name(cluster=w378, "Spliter_matrix"=w367) -> (w379:T1)
                            n158 = Replace Array Subset(array=w375, new element=w379, index=w377) -> (w374:T1[])
                          }
                          frame False {
                            n159 = Index Array(array=w392, index (row)=2, index (col)=w383) -> (element=w396:i32)
                            n160 = call "CRYSearch Matrix Element.vi"("element"=w396, "index (row)"=0, "matrix in"=w392) -> ("index of element"=w393:i32)  [unwired: 8 in]
                            n161 = local read "sp_mUp_ypos"() -> (w405:i32)
                            n162 = local read "sp_mUp_hei"() -> (w406:i32)
                            n163 = local read "sp_mUp_xpos"() -> (w389:i32)
                            n164 = local read "sp_mUp_wid"() -> (w404:i32)
                            n165 = Add(x=w405, y=w406) -> (x+y=w387:i32)
                            n166 = Index Array(array=w392, index (row) #1=7 ("index (row)"), index (col) #1=w393, index (row) #2=8 ("index (row)"), index (col) #2=w393) -> (element #1=w385:i32, element #2=w382:i32)
                            n167 = Add(x=w389, y=w404) -> ()  [unwired: 1 out]
                            n168 = Replace Array Subset(array=w392, new element #1=w389, index (row) #1=5 ("disabled index (row)"), index (col) #1=w383, new element #2=w387, index (row) #2=6 ("disabled index (row)"), index (col) #2=w383, new element #3=w385, index (row) #3=7 ("disabled index (row)"), index (col) #3=w383, new element #4=w382, index (row) #4=8 ("disabled index (row)"), index (col) #4=w383) -> (w391:i32[][])
                            n169 = Bundle By Name(cluster=w402, "Spliter_matrix"=w391) -> (w403:T1)
                            n170 = Replace Array Subset(array=w399, new element=w403, index=w401) -> (w398:T1[])
                          }
                        }
                      }
                    }
                  }
                }
              }
              frame True {
                # "Is Current Splitter Horizontal?"
                n171 = call "CRYSearch Matrix Element.vi"("element"=w411, "index (row)"=0, "matrix in"=w407) -> ("index of element"=w423:i32)  [unwired: 8 in]
                n172 = call "CRYSearch Matrix Element.vi"("element"=w411, "index (row)"=0, "matrix in"=w412) -> ("index of element"=w414:i32)  [unwired: 8 in]
                n173 = Index Array(array=w407, index (row)=1 ("disabled index (row)"), index (col)=w423) -> (element=w421:i32)
                n174 = Index Array(array=w412, index (row) #1=1 ("disabled index (row)"), index (col) #1=w414, index (row) #2=2 ("disabled index (row)"), index (col) #2=w414, index (row) #3=3 ("disabled index (row)"), index (col) #3=w414, index (row) #4=4 ("disabled index (row)"), index (col) #4=w414) -> (element #1=w409:i32, element #2=w408:i32)  [unwired: 2 out]
                n175 = Equal?(x=w421, y=1) -> (x = y?=w410:bool)
                n176 = case shown="False" w410 {
                  tunnel: w429 -> [w439 w544]
                  tunnel: w428 -> [w440 w543]
                  tunnel: w411 -> [w438 w542]
                  tunnel: w412 -> [w437 w541]
                  tunnel: w407 -> [w436 w540]
                  tunnel: w427 -> [w435 w539]
                  tunnel: w424 -> [w434 w538]
                  tunnel: w426 -> [w433 w537]
                  tunnel: [w432 w536] -> w425
                  tunnel: w409 -> [w430 w535]
                  tunnel: w408 -> [w431 _]
                  frame False {
                    n177 = stacked-sequence {
                      seq-local: [w468 _] -> [_ w488]
                      tunnel: w440 -> [w479 _]
                      tunnel: w439 -> [w461 _]
                      tunnel: w438 -> [w478 w483]
                      tunnel: w437 -> [w460 _]
                      tunnel: w436 -> [w452 w485]
                      tunnel: w435 -> [_ w487]
                      tunnel: w434 -> [_ w486]
                      tunnel: w433 -> [_ w481]
                      tunnel: [_ w480] -> w432
                      tunnel: w431 -> [w446 _]
                      tunnel: w430 -> [w445 _]
                      frame #0 {
                        n178 = local read "sp_mUp_xpos"() -> (w477:i32)
                        n179 = call "CRYSearch Matrix Element.vi"("element"=w461, "index (row)"=0, "matrix in"=w452) -> ("index of element"=w449:i32)  [unwired: 8 in]
                        n180 = call "CRYSearch Matrix Element.vi"("element"=w461, "index (row)"=0, "matrix in"=w460) -> ("index of element"=w456:i32)  [unwired: 8 in]
                        n181 = Index Array(array=w479, index=w478) -> (element=w444:refnum<vi>)
                        n182 = global read "CRYNew View Global.vi" "splitter_thickness"() -> (w441:u32)
                        n183 = local read "sp_mUp_xpos"() -> (w467:i32)
                        n184 = Index Array(array=w460, index (row) #1=1 ("index (row)"), index (col) #1=w456, index (row) #2=4 ("index (row)"), index (col) #2=w456, index (row) #3=2 ("index (row)"), index (col) #3=w456) -> (element #1=w455:i32, element #2=w454:i32, element #3=w453:i32)
                        n185 = Index Array(array=w452, index (row) #1=5 ("index (row)"), index (col) #1=w449, index (row) #2=7 ("index (row)"), index (col) #2=w449) -> (element #1=w448:i32, element #2=w447:i32)
                        n186 = Add(x=w477, y=w441) -> (x+y=w465:u32)
                        n187 = local read "sp_mUp_hei"() -> (w475:i32)
                        n188 = Subtract(x=w467, y=w448) -> (x-y=w466:i32)
                        n189 = Subtract(x=w447, y=w465) -> (x-y=w464:u32)
                        n190 = Subtract(x=w446, y=w453) -> (x-y=w474:i32)
                        n191 = Greater?(x=w455, y=w445) -> (0:w468:bool)
                        n192 = Select(t=w466, s=w468, f=w464) -> (s? t:f=w469:u32)
                        n193 = Select(t=w448, s=w468, f=w465) -> (s? t:f=w476:u32)
                        n194 = Multiply(x=w475, y=w474) -> (x*y=w473:i32)
                        n195 = local read "sp_mUp_ypos"() -> (w472:i32)
                        n196 = Divide(x=w473, y=w454) -> (x/y=w471:dbl)
                        n197 = global read "CRYNew View Global.vi" "splitter_thickness"() -> (w443:u32)
                        n198 = To Long Integer(number=w471) -> (32bit integer=w442:i32)
                        n199 = Add(x=w472, y=w442) -> (x+y=w470:i32)
                        n200 = property class="Bool"(reference=w444, "Width"=w469, "Height"=w443) -> ()  [unwired: 1 in, 2 out]
                        n201 = property class="Bool"(reference=w444, "Left"=w476, "Top"=w470) -> ()  [unwired: 1 in, 2 out]
                      }
                      frame #1 {
                        n202 = call "CRYSearch Matrix Element.vi"("element"=w483, "index (row)"=0, "matrix in"=w485) -> ("index of element"=w482:i32)  [unwired: 8 in]
                        n203 = case shown="False" w488 {
                          tunnel: w482 -> [w490 w513]
                          tunnel: w485 -> [w499 w521]
                          tunnel: w487 -> [w508 w530]
                          tunnel: w486 -> [w507 w529]
                          tunnel: w481 -> [w505 w527]
                          tunnel: [w504 w526] -> w480
                          frame True {
                            n204 = Index Array(array=w499, index (row)=2, index (col)=w490) -> (element=w502:i32)
                            n205 = call "CRYSearch Matrix Element.vi"("element"=w502, "index (row)"=0, "matrix in"=w499) -> ("index of element"=w500:i32)  [unwired: 8 in]
                            n206 = local read "sp_mUp_ypos"() -> (w495:i32)
                            n207 = local read "sp_mUp_hei"() -> (w510:i32)
                            n208 = local read "sp_mUp_xpos"() -> (w493:i32)
                            n209 = Add(x=w495, y=w510) -> (x+y=w491:i32)
                            n210 = Index Array(array=w499, index (row)=5, index (col)=w500) -> (element=w497:i32)
                            n211 = Replace Array Subset(array=w499, new element #1=w497, index (row) #1=5 ("disabled index (row)"), index (col) #1=w490, new element #2=w495, index (row) #2=6 ("disabled index (row)"), index (col) #2=w490, new element #3=w493, index (row) #3=7 ("disabled index (row)"), index (col) #3=w490, new element #4=w491, index (row) #4=8 ("disabled index (row)"), index (col) #4=w490) -> (w489:i32[][])
                            n212 = Bundle By Name(cluster=w508, "Spliter_matrix"=w489) -> (w509:T1)
                            n213 = Replace Array Subset(array=w505, new element=w509, index=w507) -> (w504:T1[])
                          }
                          frame False {
                            n214 = Index Array(array=w521, index (row)=2, index (col)=w513) -> (element=w524:i32)
                            n215 = call "CRYSearch Matrix Element.vi"("element"=w524, "index (row)"=0, "matrix in"=w521) -> ("index of element"=w522:i32)  [unwired: 8 in]
                            n216 = local read "sp_mUp_ypos"() -> (w517:i32)
                            n217 = local read "sp_mUp_xpos"() -> (w533:i32)
                            n218 = local read "sp_mUp_wid"() -> (w532:i32)
                            n219 = local read "sp_mUp_hei"() -> (w534:i32)
                            n220 = Add(x=w533, y=w532) -> (x+y=w519:i32)
                            n221 = Add(x=w517, y=w534) -> (x+y=w512:i32)
                            n222 = Index Array(array=w521, index (row)=7, index (col)=w522) -> (element=w515:i32)
                            n223 = Replace Array Subset(array=w521, new element #1=w519, index (row) #1=5 ("disabled index (row)"), index (col) #1=w513, new element #2=w517, index (row) #2=6 ("disabled index (row)"), index (col) #2=w513, new element #3=w515, index (row) #3=7 ("disabled index (row)"), index (col) #3=w513, new element #4=w512, index (row) #4=8 ("disabled index (row)"), index (col) #4=w513) -> (w511:i32[][])
                            n224 = Bundle By Name(cluster=w530, "Spliter_matrix"=w511) -> (w531:T1)
                            n225 = Replace Array Subset(array=w527, new element=w531, index=w529) -> (w526:T1[])
                          }
                        }
                      }
                    }
                  }
                  frame True {
                    n226 = stacked-sequence {
                      seq-local: [w584 _] -> [_ w598]
                      tunnel: w544 -> [w564 _]
                      tunnel: w543 -> [w589 _]
                      tunnel: w542 -> [w571 w593]
                      tunnel: w541 -> [w563 _]
                      tunnel: w540 -> [w555 w594]
                      tunnel: w539 -> [_ w597]
                      tunnel: w538 -> [_ w596]
                      tunnel: w537 -> [_ w591]
                      tunnel: [_ w590] -> w536
                      tunnel: w535 -> [w549 _]
                      frame #0 {
                        n227 = call "CRYSearch Matrix Element.vi"("element"=w564, "index (row)"=0, "matrix in"=w563) -> ("index of element"=w559:i32)  [unwired: 8 in]
                        n228 = call "CRYSearch Matrix Element.vi"("element"=w564, "index (row)"=0, "matrix in"=w555) -> ("index of element"=w552:i32)  [unwired: 8 in]
                        n229 = local read "sp_mUp_xpos"() -> (w567:i32)
                        n230 = local read "sp_mUp_xpos"() -> (w587:i32)
                        n231 = local read "sp_mUp_wid"() -> (w583:i32)
                        n232 = Index Array(array=w563, index (row) #1=1 ("index (row)"), index (col) #1=w559, index (row) #2=5 ("index (row)"), index (col) #2=w559, index (row) #3=7 ("index (row)"), index (col) #3=w559) -> (element #1=w558:i32, element #2=w557:i32, element #3=w556:i32)
                        n233 = Subtract(x=w587, y=w558) -> ()  [unwired: 1 out]
                        n234 = Subtract(x=w558, y=w557) -> (x-y=w576:i32)
                        n235 = Add(x=w567, y=w583) -> (x+y=w568:i32)
                        n236 = Add(x=w558, y=w583) -> (x+y=w569:i32)
                        n237 = Index Array(array=w589, index=w571) -> (element=w548:refnum<vi>)
                        n238 = Index Array(array=w555, index (row) #1=5 ("index (row)"), index (col) #1=w552, index (row) #2=7 ("index (row)"), index (col) #2=w552) -> (element #1=w550:i32, element #2=w551:i32)
                        n239 = Subtract(x=w567, y=w550) -> (x-y=w577:i32)
                        n240 = Subtract(x=w551, y=w568) -> (x-y=w582:i32)
                        n241 = Subtract(x=w556, y=w569) -> (x-y=w581:i32)
                        n242 = Divide(x=w577, y=w576) -> (x/y=w575:dbl)
                        n243 = Subtract(x=w549, y=w557) -> (x-y=w574:i32)
                        n244 = Greater?(x=w558, y=w549) -> (0:w584:bool)
                        n245 = Subtract(x=w549, y=w558) -> (x-y=w570:i32)
                        n246 = Divide(x=w582, y=w581) -> (x/y=w580:dbl)
                        n247 = local read "sp_mUp_hei"() -> (w588:i32)
                        n248 = Multiply(x=w575, y=w574) -> (x*y=w573:dbl)
                        n249 = Multiply(x=w580, y=w570) -> (x*y=w579:dbl)
                        n250 = global read "CRYNew View Global.vi" "splitter_thickness"() -> (w545:u32)
                        n251 = To Long Integer(number=w573) -> (32bit integer=w547:i32)
                        n252 = To Long Integer(number=w579) -> (32bit integer=w546:i32)
                        n253 = Add(x=w547, y=w550) -> (x+y=w572:i32)
                        n254 = Add(x=w546, y=w567) -> (x+y=w578:i32)
                        n255 = local read "sp_mUp_ypos"() -> (w586:i32)
                        n256 = Select(t=w572, s=w584, f=w578) -> (s? t:f=w585:i32)
                        n257 = property class="Bool"(reference=w548, "Width"=w545, "Height"=w588) -> ()  [unwired: 1 in, 2 out]
                        n258 = property class="Bool"(reference=w548, "Left"=w585, "Top"=w586) -> ()  [unwired: 1 in, 2 out]
                      }
                      frame #1 {
                        n259 = call "CRYSearch Matrix Element.vi"("element"=w593, "index (row)"=0, "matrix in"=w594) -> ("index of element"=w592:i32)  [unwired: 8 in]
                        n260 = case shown="True" w598 {
                          tunnel: w592 -> [w601 w623]
                          tunnel: w594 -> [w609 w631]
                          tunnel: w597 -> [w618 w640]
                          tunnel: w596 -> [w617 w639]
                          tunnel: w591 -> [w615 w637]
                          tunnel: [w614 w636] -> w590
                          frame True {
                            n261 = Index Array(array=w609, index (row)=2, index (col)=w601) -> (element=w612:i32)
                            n262 = call "CRYSearch Matrix Element.vi"("element"=w612, "index (row)"=0, "matrix in"=w609) -> ("index of element"=w610:i32)  [unwired: 8 in]
                            n263 = local read "sp_mUp_ypos"() -> (w605:i32)
                            n264 = local read "sp_mUp_hei"() -> (w620:i32)
                            n265 = local read "sp_mUp_xpos"() -> (w603:i32)
                            n266 = Add(x=w605, y=w620) -> (x+y=w600:i32)
                            n267 = Index Array(array=w609, index (row)=5, index (col)=w610) -> (element=w607:i32)
                            n268 = Replace Array Subset(array=w609, new element #1=w607, index (row) #1=5 ("disabled index (row)"), index (col) #1=w601, new element #2=w605, index (row) #2=6 ("disabled index (row)"), index (col) #2=w601, new element #3=w603, index (row) #3=7 ("disabled index (row)"), index (col) #3=w601, new element #4=w600, index (row) #4=8 ("disabled index (row)"), index (col) #4=w601) -> (w599:i32[][])
                            n269 = Bundle By Name(cluster=w618, "Spliter_matrix"=w599) -> (w619:T1)
                            n270 = Replace Array Subset(array=w615, new element=w619, index=w617) -> (w614:T1[])
                          }
                          frame False {
                            n271 = Index Array(array=w631, index (row)=2, index (col)=w623) -> (element=w634:i32)
                            n272 = call "CRYSearch Matrix Element.vi"("element"=w634, "index (row)"=0, "matrix in"=w631) -> ("index of element"=w632:i32)  [unwired: 8 in]
                            n273 = local read "sp_mUp_ypos"() -> (w627:i32)
                            n274 = local read "sp_mUp_xpos"() -> (w643:i32)
                            n275 = local read "sp_mUp_wid"() -> (w642:i32)
                            n276 = local read "sp_mUp_hei"() -> (w644:i32)
                            n277 = Add(x=w643, y=w642) -> (x+y=w629:i32)
                            n278 = Add(x=w627, y=w644) -> (x+y=w622:i32)
                            n279 = Index Array(array=w631, index (row)=7, index (col)=w632) -> (element=w625:i32)
                            n280 = Replace Array Subset(array=w631, new element #1=w629, index (row) #1=5 ("disabled index (row)"), index (col) #1=w623, new element #2=w627, index (row) #2=6 ("disabled index (row)"), index (col) #2=w623, new element #3=w625, index (row) #3=7 ("disabled index (row)"), index (col) #3=w623, new element #4=w622, index (row) #4=8 ("disabled index (row)"), index (col) #4=w623) -> (w621:i32[][])
                            n281 = Bundle By Name(cluster=w640, "Spliter_matrix"=w621) -> (w641:T1)
                            n282 = Replace Array Subset(array=w637, new element=w641, index=w639) -> (w636:T1[])
                          }
                        }
                      }
                    }
                  }
                }
              }
            }
          }
          frame #1 {
            n283 = Index Array(array=w645, index=w648) -> (element=w649:T1)
            n284 = Unbundle By Name(w649) -> ("Spliter_matrix"=w646:i32[][], "Panel_matrix"=w647:i32[][])
            n285 = while {
              shift-right: [w654] -> _
              shift-left: -1 -> [w657]
              tunnel: w653 -> [w655]
              tunnel: w652 -> [w664]
              tunnel: w651 -> [w663]
              tunnel: w647 -> [w659]
              tunnel: w646 -> [w660]
              stop <- w662 stop-if-true
              n286 = Increment(x=w657) -> (x+1=w656:i32)
              n287 = call "CRYSearch Matrix Element.vi"("start index"=w656, "element"=w655, "index (row)"=0, "matrix in"=w659) -> ("index of element"=w654:i32)  [unwired: 7 in]
              n288 = Less Than 0?(x=w654) -> (x < 0?=w662:bool)
              n289 = Not(x=w662) -> (.not. x?=w661:bool)
              n290 = case shown="True" w661 {
                tunnel: w654 -> [_ w678]
                tunnel: w664 -> [_ w685]
                tunnel: w663 -> [_ w687]
                tunnel: w655 -> [_ w682]
                tunnel: w660 -> [_ w670]
                tunnel: w659 -> [_ w679]
                frame False {
                }
                frame True {
                  n291 = stacked-sequence {
                    tunnel: w687 -> [w689]
                    tunnel: w682 -> [w690]
                    tunnel: [w689] -> w686
                    frame #0 {
                      n292 = Index Array(array=w689, index=w690) -> (element=w688:refnum<vi>)
                      n293 = property class="Bool"(reference=w688) -> ("Left"=w694:i32, "Top"=w693:i32)  [unwired: 1 in, 2 out]
                      n294 = local write "cur_sp_xpos"(w694) -> ()
                      n295 = local write "cur_sp_ypos"(w693) -> ()
                      n296 = property class="Bool"(reference=w688) -> ("Height"=w692:u32, "Width"=w691:u32)  [unwired: 1 in, 2 out]
                      n297 = local write "cur_sp_hei"(w692) -> ()
                      n298 = local write "cur_sp_wid"(w691) -> ()
                    }
                  }
                  n299 = Index Array(array=w679, index (row) #1=1 ("index (row)"), index (col) #1=w678, index (row) #2=2 ("index (row)"), index (col) #2=w678) -> (element #1=w677:i32, element #2=w676:i32)
                  n300 = Index Array(array=w685, index=w677) -> (element=w684:refnum<vi>)
                  n301 = call "CRYSearch Matrix Element.vi"("element"=w682, "index (row)"=0, "matrix in"=w670) -> ("index of element"=w671:i32)  [unwired: 8 in]
                  n302 = Index Array(array=w670, index (row) #1=5 ("index (row)"), index (col) #1=w671, index (row) #2=6 ("index (row)"), index (col) #2=w671, index (row) #3=7 ("index (row)"), index (col) #3=w671, index (row) #4=8 ("index (row)"), index (col) #4=w671) -> (element #1=w669:i32, element #2=w668:i32, element #3=w667:i32, element #4=w666:i32)
                  n303 = global read "CRYNew View Global.vi" "panel_offset"() -> (w665:i32)
                  n304 = case shown="4" w676 {
                    tunnel: w669 -> [_ w702 _ w719 w723]
                    tunnel: w668 -> [_ w703 w711 w716 _]
                    tunnel: w667 -> [_ _ w710 _ _]
                    tunnel: w666 -> [_ _ _ _ w727]
                    tunnel: w686 -> [_ _ _ _ _]
                    tunnel: w684 -> [_ w698 w714 w720 w731]
                    tunnel: w665 -> [_ w695 w704 _ w721]
                    frame 0, Default {
                    }
                    frame 1 {
                      n305 = local read "cur_sp_xpos"() -> (w701:i32)
                      n306 = local read "cur_sp_hei"() -> (w699:i32)
                      n307 = Subtract(x=w702, y=w695) -> (x-y=w697:i32)
                      n308 = Subtract(x=w701, y=w702) -> (x-y=w700:i32)
                      n309 = Subtract(x=w703, y=w695) -> (x-y=w696:i32)
                      n310 = property class="SubPnl"(reference=w698, "Width"=w700, "Height"=w699, "Left"=w697, "Top"=w696) -> ()  [unwired: 1 in, 2 out]
                    }
                    frame 2 {
                      n311 = local read "cur_sp_xpos"() -> (w713:i32)
                      n312 = local read "cur_sp_wid"() -> (w712:i32)
                      n313 = Add(x=w713, y=w712) -> (x+y=w709:i32)
                      n314 = local read "cur_sp_hei"() -> (w707:i32)
                      n315 = Subtract(x=w710, y=w709) -> (x-y=w708:i32)
                      n316 = Subtract(x=w711, y=w704) -> (x-y=w705:i32)
                      n317 = Subtract(x=w709, y=w704) -> (x-y=w706:i32)
                      n318 = property class="SubPnl"(reference=w714, "Width"=w708, "Height"=w707, "Left"=w706, "Top"=w705) -> ()  [unwired: 1 in, 2 out]
                    }
                    frame 3 {
                      n319 = local read "cur_sp_ypos"() -> (w717:i32)
                      n320 = local read "cur_sp_wid"() -> (w718:i32)
                      n321 = Subtract(x=w717, y=w716) -> (x-y=w715:i32)
                      n322 = property class="SubPnl"(reference=w720, "Width"=w718, "Height"=w715, "Left"=w719, "Top"=w716) -> ()  [unwired: 1 in, 2 out]
                    }
                    frame 4 {
                      n323 = local read "cur_sp_ypos"() -> (w729:i32)
                      n324 = local read "cur_sp_hei"() -> (w728:i32)
                      n325 = Add(x=w729, y=w728) -> (x+y=w726:i32)
                      n326 = local read "cur_sp_wid"() -> (w730:i32)
                      n327 = Subtract(x=w727, y=w726) -> (x-y=w725:i32)
                      n328 = Subtract(x=w723, y=w721) -> (x-y=w724:i32)
                      n329 = Subtract(x=w726, y=w721) -> (x-y=w722:i32)
                      n330 = property class="SubPnl"(reference=w731, "Width"=w730, "Height"=w725, "Left"=w724, "Top"=w722) -> ()  [unwired: 1 in, 2 out]
                    }
                  }
                }
              }
            }
          }
        }
      }
    }
  }
  n331 = global write "CRYNew View Global.vi" "DataView_Global"(w6) -> ()
